vi "GetDigitalFilterCount.vi"(8 "Error In":errorcluster, 10 "Channel (1 or 2)":u8 min=1 max=2 step=1, 11 "Keithley 6482 In":refnum<visa-resource-name>) -> (0 "Error Out":errorcluster, 2 "Count (1-100)":u8, 3 "Keithley 6482 Out":refnum<visa-resource-name>)   [LabVIEW 2009, in "Keithley-6482-Visa.lvlib"]
uses:
  <instrlib>/Keithley-6482-Visa9.0/Keithley-6482-Visa.lvlib
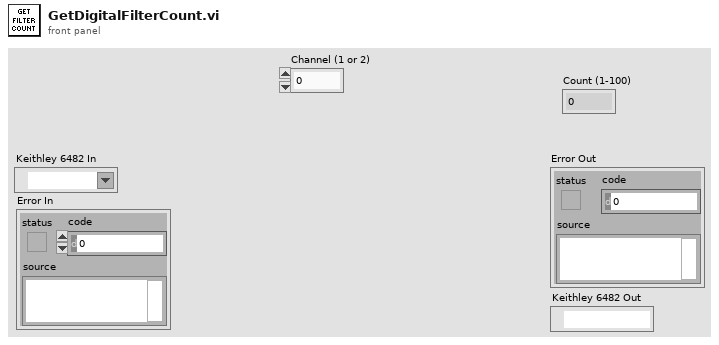
[diagram p1: front panel]
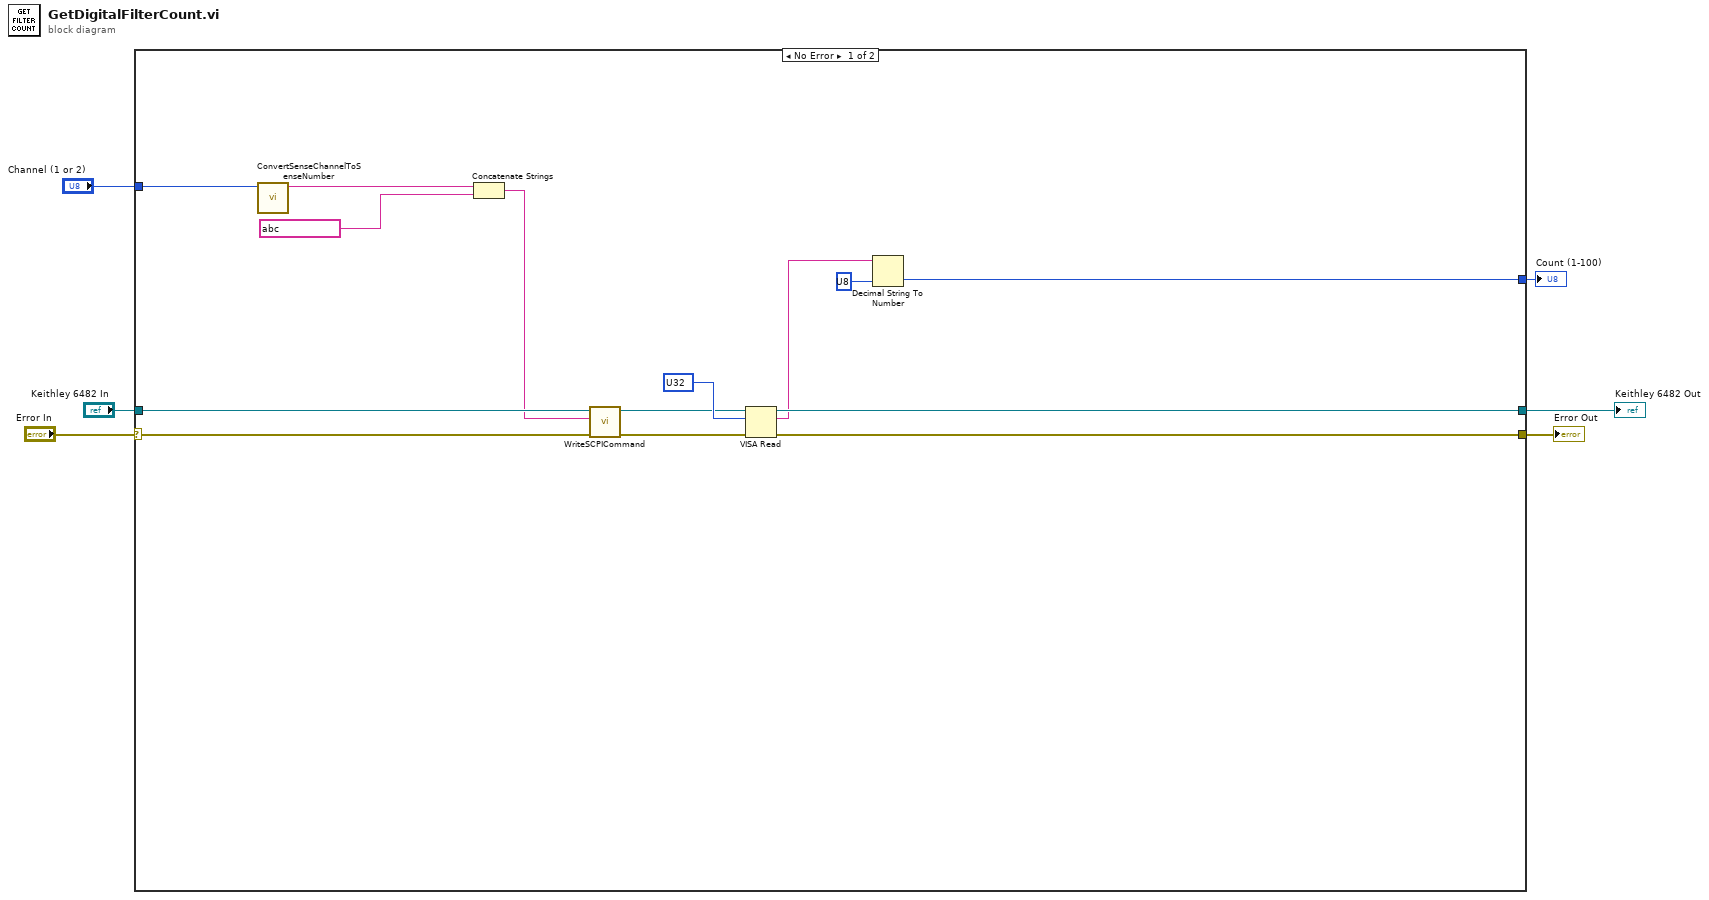
[diagram p0: block diagram]
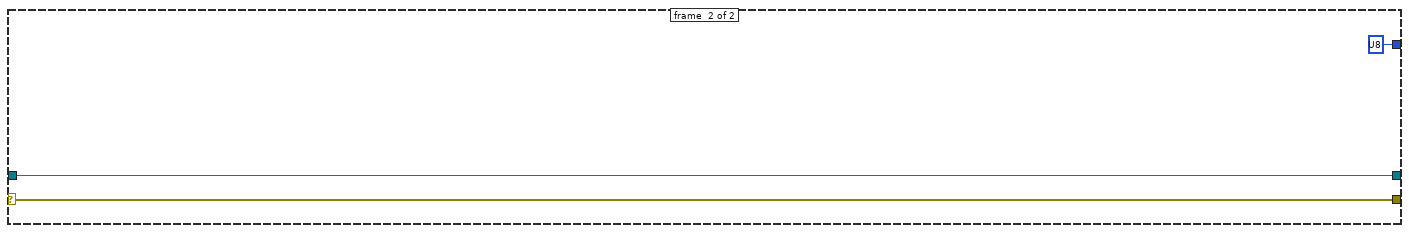
[diagram p2: hidden frame]
diagram:
  n1 = case shown="No Error" "Error In" {
    selector: "Error In" -> [w15 w22]
    tunnel: "Keithley 6482 In" -> [w14 w23]
    tunnel: [w20 w22] -> w4
    tunnel: [w19 w23] -> w3
    tunnel: "Channel (1 or 2)" -> [w13 _]
    tunnel: [w7 u8 ?] -> w1
    frame #0 {
      n2 = call <instrlib>:"ConvertSenseChannelToSenseNumber.vi"("Channel (1 or 2)"=w13) -> ("Sense Number"=w12:string)  [unwired: 10 in]
      n3 = Concatenate Strings(w12, string ? ("string")) -> (w10:string)
      n4 = call <instrlib>:"WriteSCPICommand.vi"("Error In"=w15, "SCPI Command"=w10, "Keithley 6482 In"=w14) -> ("Error Out"=w16:errorcluster, "Keithley 6482 Out"=w17:refnum<visa-resource-name>)  [unwired: 7 in]
      n5 = VISA Read(VISA resource name=w17, byte count=u32 ?, error in (no error)=w16) -> (VISA resource name out=w19:refnum<visa-resource-name>, read buffer=w9:string, error out=w20:errorcluster)  [unwired: 1 out]
      n6 = Decimal String To Number(string=w9, default (0L)=u8 ?) -> (number=w7:u8)  [unwired: 1 in, 1 out]
    }
    frame #1 {
    }
  }
  "Error Out" <- w4
  "Keithley 6482 Out" <- w3
  "Count (1-100)" <- w1
